vi "matlab-for-complementary-filter.vi"(0 "Acceleration Data (g)":T1, 1 "Gyro  Data (dps)":T1, 4 "PLRESET":dbl, 5 "error in (no error)":errorcluster) -> (12 "y_pos":dbl, 14 "angle_y":dbl, 16 "Path Length":dbl, 17 "angle_x":dbl, 18 "x_pos":dbl, 19 "error out":errorcluster)   [LabVIEW 2016]
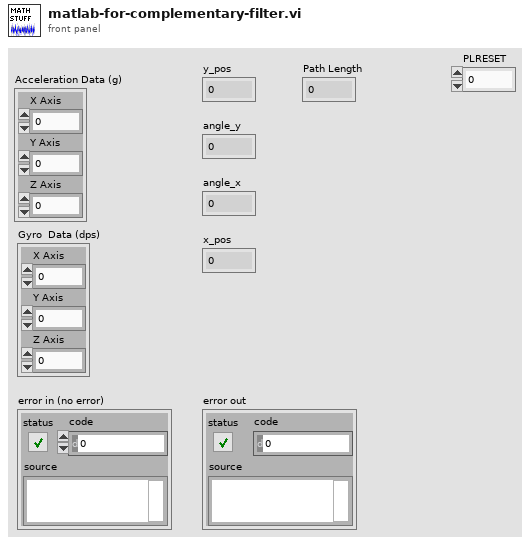
[diagram p1: front panel]
types:
  T1 = cluster{"X Axis":i16, "Y Axis":i16, "Z Axis":i16}
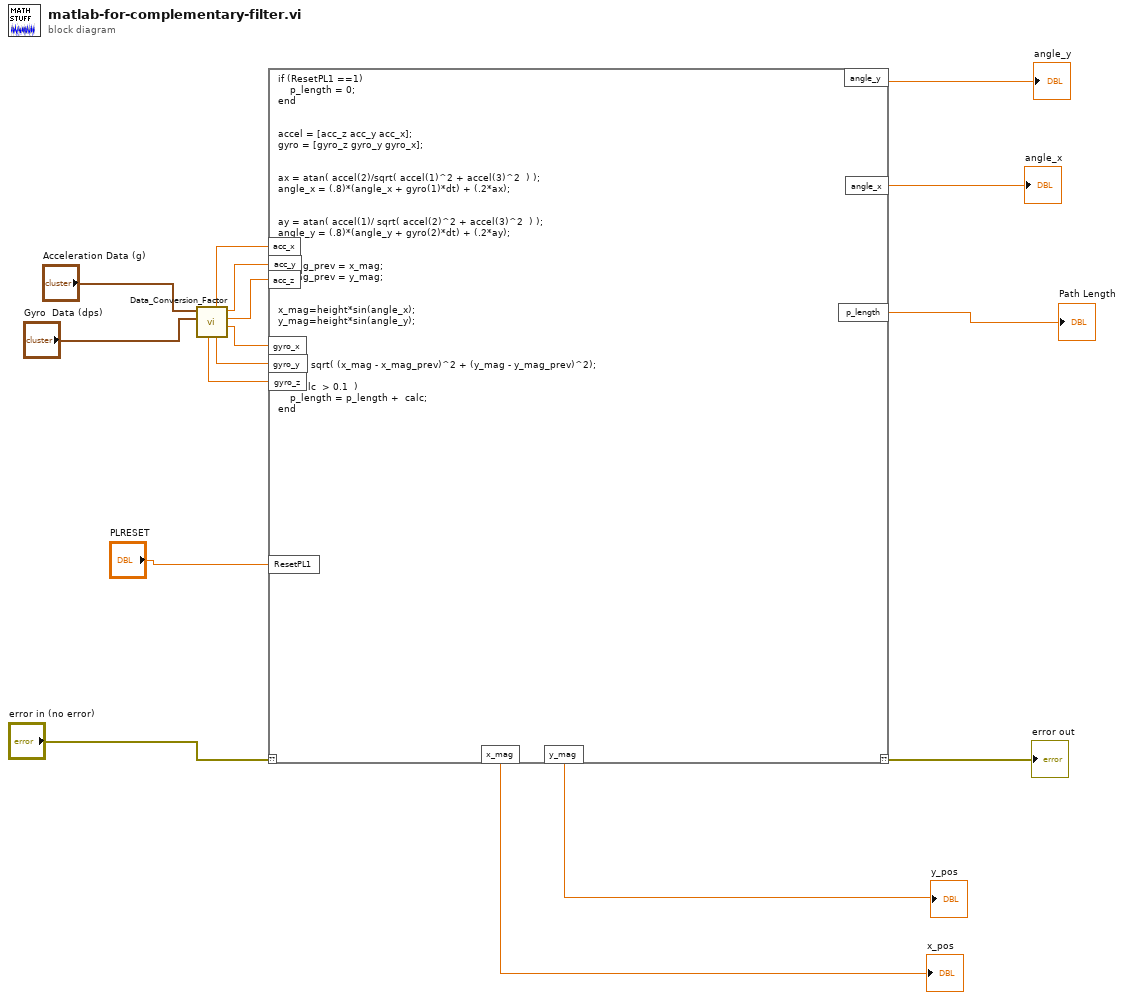
[diagram p0: block diagram]
diagram:
  n1 = call "Data_Conversion_Factor.vi"("Gyro  Data (dps)"="Gyro  Data (dps)", "Acceleration Data (g)"="Acceleration Data (g)") -> ("Gyro_X"=w11:dbl, "Accel_Z"=w10:dbl, "Accel_Y"=w9:dbl, "Gyro_Y"=w12:dbl, "Accel_X"=w8:dbl, "Gyro_Z"=w13:dbl)  [unwired: 4 in]
  n2 = script code="if (ResetPL1 ==1) \n    p_length = 0;\nend\n\n\naccel = [acc_z acc_y acc_x];\ngyro = [gyro_z gyro_y gyro_x];\n\n\nax = atan( accel(2)/sqrt( accel(1)^2 + accel(3)^2  ) );\nangle_x = (.8)*(angle_x + gyro(1)*dt) + (.2*ax);\n\n\nay = atan( accel(1)/ sqrt( accel(2)^2 + accel(3)^2  ) );\nangle_y = (.8)*(angle_y + gyro(2)*dt) + (.2*ay);\n\n\nx_mag_prev = x_mag;\ny_mag_prev = y_mag;\n\n\nx_mag=height*sin(angle_x); \ny_mag=height*sin(angle_y);\n\n\n\ncalc = sqrt( (x_mag - x_mag_prev)^2 + (y_mag - y_mag_prev)^2);\n\nif (  calc  > 0.1  ) \n    p_length = p_length +  calc;\nend"("??"="error in (no error)", "acc_y"=w9, "acc_z"=w10, "gyro_x"=w11, "gyro_y"=w12, "gyro_z"=w13, "acc_x"=w8, "ResetPL1"="PLRESET") -> ("??"=→"error out":errorcluster, "angle_y"=→"angle_y":dbl, "angle_x"=→"angle_x":dbl, "x_mag"=→"x_pos":dbl, "y_mag"=→"y_pos":dbl, "p_length"=→"Path Length":dbl)
